vi "selectTrigger.vi"(4 "MCSSelectTrigger":T1) -> (1 "Boolean":bool)   [LabVIEW 2014]
uses:
  Controls/MCSselectRigger.ctl
  <vilib>/rvi/eio/common/nirviEmuTemplateMethod_errors.vi
  <vilib>/eio/EIONode/EIONode.xnode
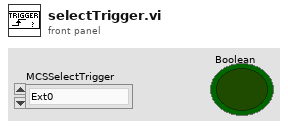
[diagram p1: front panel]
types:
  T1 = typedef "MCSselectRigger.ctl" = enum8{"Ext0", "Ext1", "Ext2", "Ext3", "Ext4", "Ext5", "Ext6", "Ext7", "Int0", "Int1", "Int2", "Int3", "Int4", "Int5", "Int6", "Int7"}
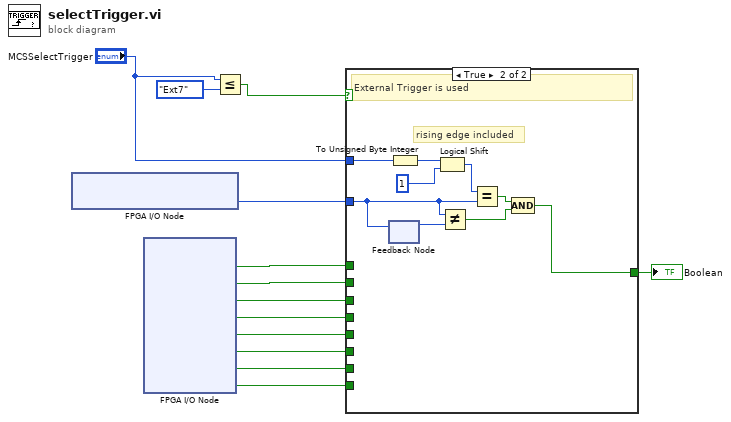
[diagram p0: block diagram]
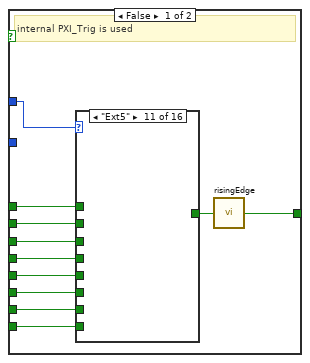
[diagram p2: hidden frame]
diagram:
  n1 = xnode "FPGA I/O Node"() -> ("Connector1/DIOPORT3"=w13:u8)  [unwired: 1 in, 1 out]
  n2 = xnode "FPGA I/O Node"() -> ("PXI_Trig0"=w12:bool, "PXI_Trig1"=w11:bool, "PXI_Trig2"=w10:bool, "PXI_Trig3"=w9:bool, "PXI_Trig4"=w8:bool, "PXI_Trig5"=w7:bool, "PXI_Trig6"=w6:bool, "PXI_Trig7"=w5:bool)  [unwired: 8 in, 8 out]
  n3 = Less Or Equal?(x="MCSSelectTrigger", y=MCSselectRigger."Ext7") -> (x <= y?=w3:bool)
  n4 = case shown="True" w3 {
    tunnel: w13 -> [_ w35]
    tunnel: w12 -> [w23 _]
    tunnel: w11 -> [w21 _]
    tunnel: w10 -> [w20 _]
    tunnel: w9 -> [w19 _]
    tunnel: w8 -> [w18 _]
    tunnel: w7 -> [w17 _]
    tunnel: w6 -> [w16 _]
    tunnel: w5 -> [w15 _]
    tunnel: "MCSSelectTrigger" -> [w24 w39]
    tunnel: [w14 w33] -> w1
    frame False {
      # "internal PXI_Trig is used"
      n5 = case shown="\"Ext5\"" w24 {
        tunnel: w23 -> [w25 _ _ _ _ _ _ _ _ _ _ _ _ _ _ _]
        tunnel: [w25 w26 w27 w28 w29 w30 w31 w32 _ _ _ _ _ _ _ _] -> w22
        tunnel: w21 -> [_ w26 _ _ _ _ _ _ _ _ _ _ _ _ _ _]
        tunnel: w20 -> [_ _ w27 _ _ _ _ _ _ _ _ _ _ _ _ _]
        tunnel: w19 -> [_ _ _ w28 _ _ _ _ _ _ _ _ _ _ _ _]
        tunnel: w18 -> [_ _ _ _ w29 _ _ _ _ _ _ _ _ _ _ _]
        tunnel: w17 -> [_ _ _ _ _ w30 _ _ _ _ _ _ _ _ _ _]
        tunnel: w16 -> [_ _ _ _ _ _ w31 _ _ _ _ _ _ _ _ _]
        tunnel: w15 -> [_ _ _ _ _ _ _ w32 _ _ _ _ _ _ _ _]
        frame "Int0" {
        }
        frame "Int1" {
        }
        frame "Int2" {
        }
        frame "Int3" {
        }
        frame "Int4" {
        }
        frame "Int5" {
        }
        frame "Int6" {
        }
        frame "Int7" {
        }
        frame "Ext7" {
        }
        frame "Ext6" {
        }
        frame "Ext5" {
        }
        frame "Ext4" {
        }
        frame "Ext3" {
        }
        frame "Ext2" {
        }
        frame "Ext1" {
        }
        frame "Ext0" {
        }
      }
      n6 = call "risingEdge.vi"("In"=w22) -> ("out"=w14:bool)
    }
    frame True {
      # "rising edge included"
      # "External Trigger is used"
      n7 = feedback-in #1(w35) -> ()
      n8 = feedback #1() -> (w36:u8)  [unwired: 1 in]
      n9 = To Unsigned Byte Integer(number=w39) -> (unsigned 8bit integer=w41:u8)
      n10 = Logical Shift(y=w41, x=u8 1) -> (x << y=w40:u8)
      n11 = Not Equal?(x=w35, y=w36) -> (x != y?=w34:bool)
      n12 = Equal?(x=w40, y=w35) -> (x = y?=w37:bool)
      n13 = Compound Arithmetic op=AND(w37, w34) -> (w33:bool)
    }
  }
  "Boolean" <- w1
